vi "Log Data.vi"(7 "FIFO Buffers":refnum<k33>[](array[refnum]), 8 "error in (no error)":errorcluster, 10 "Fault Index":i32, 11 "Refnum in":refnum<k34>) -> (0 "error out":errorcluster, 3 "Refnum out":refnum<k34>)   [LabVIEW 2014]
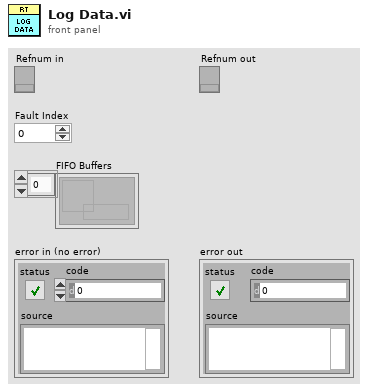
[diagram p1: front panel]
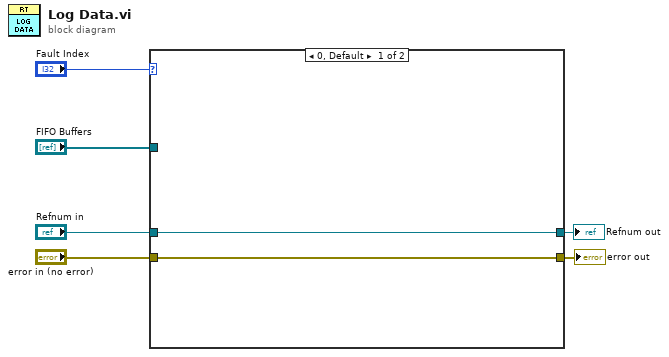
[diagram p0: block diagram]
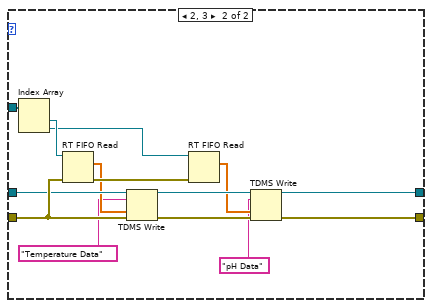
[diagram p2: hidden frame]
diagram:
  n1 = case shown="0, Default" "Fault Index" {
    tunnel: "error in (no error)" -> [w7 w20]
    tunnel: "FIFO Buffers" -> [_ w19]
    tunnel: "Refnum in" -> [w8 w15]
    tunnel: [w8 w14] -> w5
    tunnel: [w7 w13] -> w6
    frame 0, Default {
    }
    frame 2, 3 {
      n2 = Index Array(array=w19) -> (element #1=w18:refnum<k33>, element #2=w17:refnum<k33>)  [unwired: 2 in]
      n3 = RT FIFO Read(0:w18, 3:w20) -> (9:w12:dbl[], 11:w22:errorcluster)  [unwired: 2 in, 3 out]
      n4 = TDMS Write(0:w15, 5:"Temperature Data" ("group name in (Untitled)"), 9:w12, 11:w20) -> (4:w16:refnum<k34>, 15:w21:errorcluster)  [unwired: 2 in, 2 out]
      n5 = RT FIFO Read(0:w17, 3:w22) -> (9:w11:dbl[])  [unwired: 2 in, 4 out]
      n6 = TDMS Write(0:w16, 5:"pH Data" ("group name in (Untitled)"), 9:w11, 11:w21) -> (4:w14:refnum<k34>, 15:w13:errorcluster)  [unwired: 2 in, 2 out]
    }
  }
  "Refnum out" <- w5
  "error out" <- w6
